vi "util_stack_dump.vi"(8 "error in (no error)":errorcluster, 11 "Lua in":refnum<class "Lua.lvclass">) -> (0 "error out":errorcluster, 2 "stack":string[](array[string]), 3 "Lua out":refnum<class "Lua.lvclass">)   [LabVIEW 2020, in "Lua for LabVIEW.lvlib" / "Lua.lvclass"]
doc: "Dump the stack to an an array of strings."
uses:
  Lua.lvclass
  Lua.lvclass/Lua.ctl
  lib/lua.dll/types/lua_error_code_offset.vi
  lib/lua.dll/lua_type.vi
  lib/lua.dll/luaL_typename.vi
  lib/lua.dll/lua_tostring.vi
  lib/lua.dll/lua_toboolean.vi
  lib/lua.dll/lua_tonumber.vi
  lib/lua.dll/lua_typename.vi
  lib/lua.dll/lua_tolstring.vi
  <vilib>/Utility/error.llb/Error Cluster From Error Code.vi
  lib/lua.dll/lua_gettop.vi
  lib/lua.dll/lua.dll.lvlib
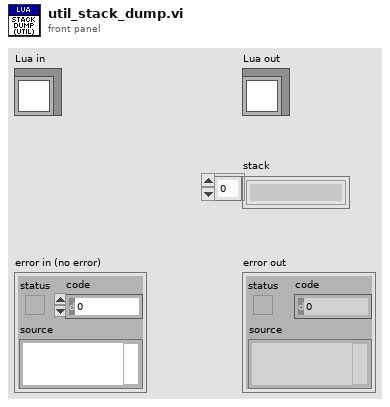
[diagram p1: front panel]
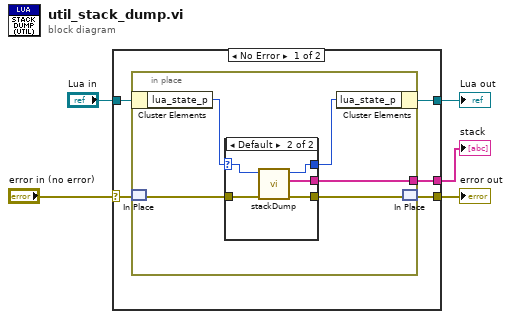
[diagram p0: block diagram]
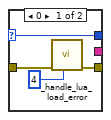
[diagram p2: hidden frame]
diagram:
  n1 = case shown="No Error" "error in (no error)" {
    selector: "error in (no error)" -> [w7 w26]
    tunnel: [w8 w26] -> w2
    tunnel: [w9 w25] -> w3
    tunnel: "Lua in" -> [w10 w25]
    tunnel: [w6 _] -> w1
    frame No Error {
      n2 = in-place {
        in-place-border: [w11] -> w6
        n3 = in-place-cluster #1(w10) -> ("lua_state_p"=w14:u64)
        n4 = in-place-match #2(w7) -> (w13:errorcluster)
        n5 = case shown="Default" w14 {
          selector: w14 -> [w19 w24]
          tunnel: [w19 w23] -> w15
          tunnel: w13 -> [w16 w21]
          tunnel: [w17 w22] -> w12
          tunnel: [_ w20] -> w11
          frame 0 {
            n6 = call "_handle_lua_load_error.vi"("lua_load errcode"=4, "error in (no error)"=w16) -> ("error out"=w17:errorcluster)  [unwired: 9 in]
          }
          frame Default {
            n7 = call "stackDump.vi"("error in (no error)"=w21, "lua_state_p"=w24) -> ("error out"=w22:errorcluster, "stack"=w20:string[], "lua_state_p out"=w23:u64)  [unwired: 7 in]
          }
        }
        n8 = in-place-cluster #1("lua_state_p"=w15) -> (w9:refnum<class "Lua.lvclass">)
        n9 = in-place-match #2(w12) -> (w8:errorcluster)
      }
    }
    frame Error {
    }
  }
  "error out" <- w2
  "Lua out" <- w3
  "stack" <- w1
